vi "Table Initialize_Str.vi"(4 "행의 개수":u32, 5 "Table Ref":refnum<vi>, 6 "Value":string, 7 "비활성화?":bool, 8 "에러 입력":errorcluster caption="에러 입력(에러 없음)", 9 "열해더 문자열":string[](array[string]), 10 "열의 개수":u32, 11 "최상단보기?":bool) -> (0 "에러 출력":errorcluster, 1 "Bottom":i32, 3 "Table Ref out":refnum<vi>)   [LabVIEW 2020]
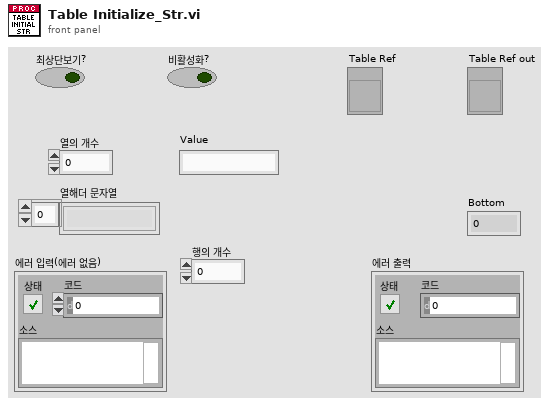
[diagram p1: front panel]
types:
  T1 = enum8{"Enabled", "Disabled", "Disabled and Grayed Out"}
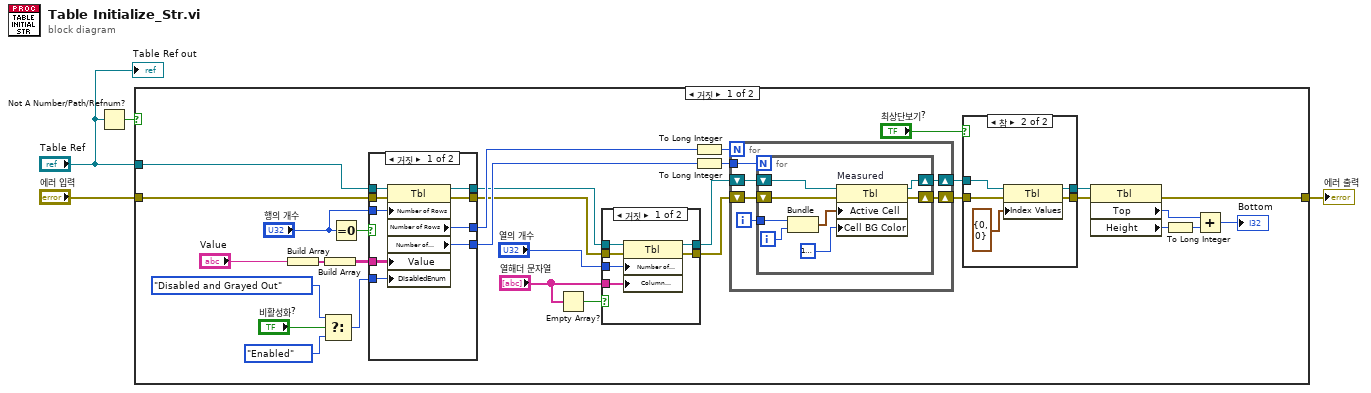
[diagram p0: block diagram]
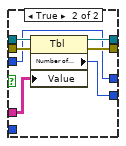
[diagram p4: hidden frame]
diagram:
  n1 = Not A Number/Path/Refnum?(number/path/refnum="Table Ref") -> (NaN/Path/Refnum?=w1:bool)
  n2 = case shown="거짓" w1 {
    tunnel: "에러 입력" -> [w34 w80]
    tunnel: "Table Ref" -> [w28 _]
    tunnel: [w22 w80] -> w3
    frame False {
      n3 = Build Array("Value") -> (w6:string[])
      n4 = Select(t=T1."Disabled and Grayed Out" ("비활성화"), s="비활성화?", f=T1."Enabled" ("비활성화")) -> (s? t:f=w14:T1)
      n5 = Build Array(w6) -> (w5:string[][])
      n6 = Equal To 0?(x="행의 개수") -> (x = 0?=w26:bool)
      n7 = case shown="거짓" w26 {
        tunnel: w34 -> [w58 w65]
        tunnel: w5 -> [w57 w64]
        tunnel: [w56 w63] -> w11
        tunnel: [w55 w62] -> w32
        tunnel: [w54 w61] -> w10
        tunnel: [w53 w59] -> w29
        tunnel: w28 -> [w52 w60]
        tunnel: "행의 개수" -> [w51 w59]
        tunnel: w14 -> [w50 _]
        frame False {
          n8 = property class="Tbl"(reference=w52, error in=w58, "Number of Rows"=w51, "Value"=w57, "DisabledEnum"=w50) -> (reference out=w54:refnum<vi>, error out=w56:errorcluster, "Number of Rows"=w53:u32, "Number of Columns"=w55:u32)
        }
        frame True {
          n9 = property class="Tbl"(reference=w60, error in=w65, "Value"=w64) -> (reference out=w61:refnum<vi>, error out=w63:errorcluster, "Number of Columns"=w62:u32)
        }
      }
      n10 = Empty Array?(array="열해더 문자열") -> (empty?=w7:bool)
      n11 = case shown="거짓" w7 {
        tunnel: w11 -> [w40 w41]
        tunnel: [w39 w41] -> _
        tunnel: [w38 w42] -> _
        tunnel: w10 -> [w37 w42]
        tunnel: "열의 개수" -> [w36 _]
        tunnel: "열해더 문자열" -> [w35 _]
        frame False {
          n12 = property class="Tbl"(reference=w37, error in=w40, "Number of Columns"=w36, "Column Headers[]"=w35) -> (reference out=w38:refnum<vi>, error out=w39:errorcluster)
        }
        frame True {
        }
      }
      n13 = To Long Integer(number=w29) -> (32bit integer=w31:i32)
      n14 = To Long Integer(number=w32) -> (32bit integer=w30:i32)
      n15 = for {
        N: w31 -> [_]
        shift-right: [w69] -> w25
        shift-left: w11 -> [w70]
        tunnel: w30 -> [w67]
        shift-right: [w66] -> w23
        shift-left: w10 -> [w71]
        i -> [w68]
        n16 = for {
          N: w67 -> [_]
          shift-right: [w77] -> w69
          shift-left: w70 -> [w78]
          tunnel: w68 -> [w76]
          shift-right: [w72] -> w66
          shift-left: w71 -> [w79]
          i -> [w75]
          n17 = Bundle(w76, w75) -> (w74:cluster{i32, i32})  [unwired: 1 in]
          n18 = property on="Measured" class="Tbl"(reference=w79, error in=w78, "Active Cell"=w74, "Cell BG Color"=u32 16777226) -> (reference out=w72:refnum<vi>, error out=w77:errorcluster)
        }
      }
      n19 = case shown="참" "최상단보기?" {
        tunnel: w25 -> [w44 w49]
        tunnel: [w44 w48] -> w13
        tunnel: w23 -> [w43 w47]
        tunnel: [w43 w45] -> w12
        frame False {
        }
        frame True {
          n20 = property class="Tbl"(reference=w47, error in=w49, "Index Values"=cluster{"Row":u32, "Column":u32} {"Row"=0, "Column"=0} ("인덱스 값")) -> (reference out=w45:refnum<vi>, error out=w48:errorcluster)
        }
      }
      n21 = property class="Tbl"(reference=w12, error in=w13) -> (error out=w22:errorcluster, "Top"=w20:i32, "Height"=w19:u32)  [unwired: 1 out]
      n22 = To Long Integer(number=w19) -> (32bit integer=w21:i32)
      n23 = Add(x=w20, y=w21) -> (x+y=→"Bottom":i32)
    }
    frame True {
    }
  }
  "에러 출력" <- w3
  "Table Ref out" <- "Table Ref"
